vi "Autonomous Independentold.vi"() -> ()   [LabVIEW 2014]
doc: "This VI is called when autonomous begins, and will automatically be terminated when autonomous ends. You can carry out timed or sensor driven robot movement independently without needing to return to the caller."
uses:
  <vilib>/Rock Robotics/WPI/Joystick/WPI_JoystickGetSetRefNum.vi
  <vilib>/Rock Robotics/Network Tables/SD Write Numeric Array.vi
  <vilib>/Rock Robotics/WPI/RobotDrive/WPI_RobotDriveMecanumDrive_Cartesian.vi
  <vilib>/Rock Robotics/Network Tables/SD Write String.vi
panel:
  in  "error in":errorcluster
  out "error out":errorcluster
  in  "error in":errorcluster
  out "error out":errorcluster
  out "error out":errorcluster
  in  "error in":errorcluster
  in  "stop":bool
  out "Current Movement, for debugging":T1 {"Z Joystick Value" scale=-1.0..1.0; "Y Joystick Value" scale=1.0..-1.0; "X Joystick Value" scale=-1.0..1.0}
  in  "Array of robot movements":T2(array[cluster]) {"Z Joystick Value" scale=-1.0..1.0; "Y Joystick Value" scale=1.0..-1.0; "X Joystick Value" scale=-1.0..1.0}
  # "Be sure to right-click and choose Data Operations>>Make Current Value default if you want to save the array values with the VI"
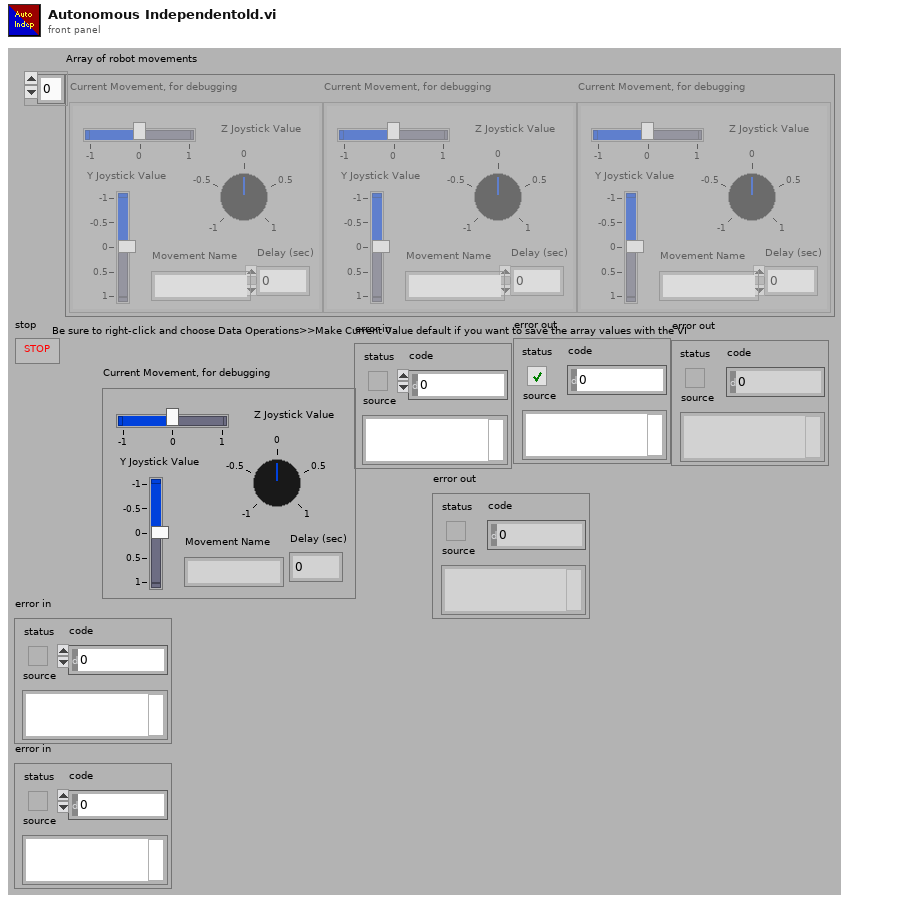
[diagram p1: front panel]
types:
  T1 = cluster{"X Joystick Value":dbl, "Y Joystick Value":dbl, "Z Joystick Value":dbl, "Delay (sec)":dbl, "Movement Name":string}
  T2 = cluster{"X Joystick Value":dbl, "Y Joystick Value":dbl, "Z Joystick Value":dbl, "Delay (sec)":dbl, "Movement Name":string}[]
  T3 = typedef "WPI_JoystickDevRef.ctl" = cluster{"Device":T4}
  T4 = typedef "WPI_JoystickDeviceEnum.ctl" = enum16{"USB 0", "USB 1", "USB 2", "USB 3", "USB 4", "USB 5"}
  T5 = typedef "WPI_RobotDriveDevRef.ctl" = cluster{"DevStatus":errorcluster, "Motors[]":T6[], "Square Inputs":bool, "Max Output":dbl}
  T6 = typedef "WPI_MotorControlDeviceRef.ctl" = cluster{"DeviceStatus":errorcluster, "Type":T7, "PWM":cluster{"Controller":T8, "PWM Channel":T9, "DeadBand":T10}, "CAN":cluster{"Device Number":u8, "Control Mode":T11, "Semaphore":T12, "Max Vout":dbl, "TalonSRX Control Mode":T13}, "Invert":bool, "TransformRef":T14, "InvTransformRef":T14}
  T7 = typedef "WPI_MotorControlType.ctl" = enum16{"PWM", "CAN", "CANTalonSRX"}
  T8 = typedef "FPGA_TypedefDigitalModule.ctl" = enum16{"Controller 1"}
  T9 = typedef "FPGA_DIOPWMChannel.ctl" = enum8{"PWM 0", "PWM 1", "PWM 2", "PWM 3", "PWM 4", "PWM 5", "PWM 6", "PWM 7", "PWM 8", "PWM 9", "PWM MXP 0", "PWM MXP 1", "PWM MXP 2", "PWM MXP 3", "PWM MXP 4", "PWM MXP 5", "PWM MXP 6", "PWM MXP 7", "PWM MXP 8", "PWM MXP 9", "Invalid"}
  T10 = typedef "WPI_PWMDeadband.ctl" = cluster{"Name":string, "maxPositivePwm":i32, "minPositivePwm":i32, "centerPwm":i32, "maxNegativePwm":i32, "minNegativePwm":i32, "angularRange":u16}
  T11 = typedef "WPI_CANJaguar_ControlMode.ctl" = enum8{"Percent VBus", "Current", "Speed", "Position", "Voltage"}
  T12 = typedef "Semaphore RefNum" = refnum<k1>
  T13 = typedef "WPI_CANTalonSRX_APIControlMode.ctl" = enum8{"Percent VBus", "Speed", "Position", "Slave", "Unchanged / Invalid"}
  T14 = typedef "WPI_PWMTransform_ConPane.ctl" = refnum<vi>
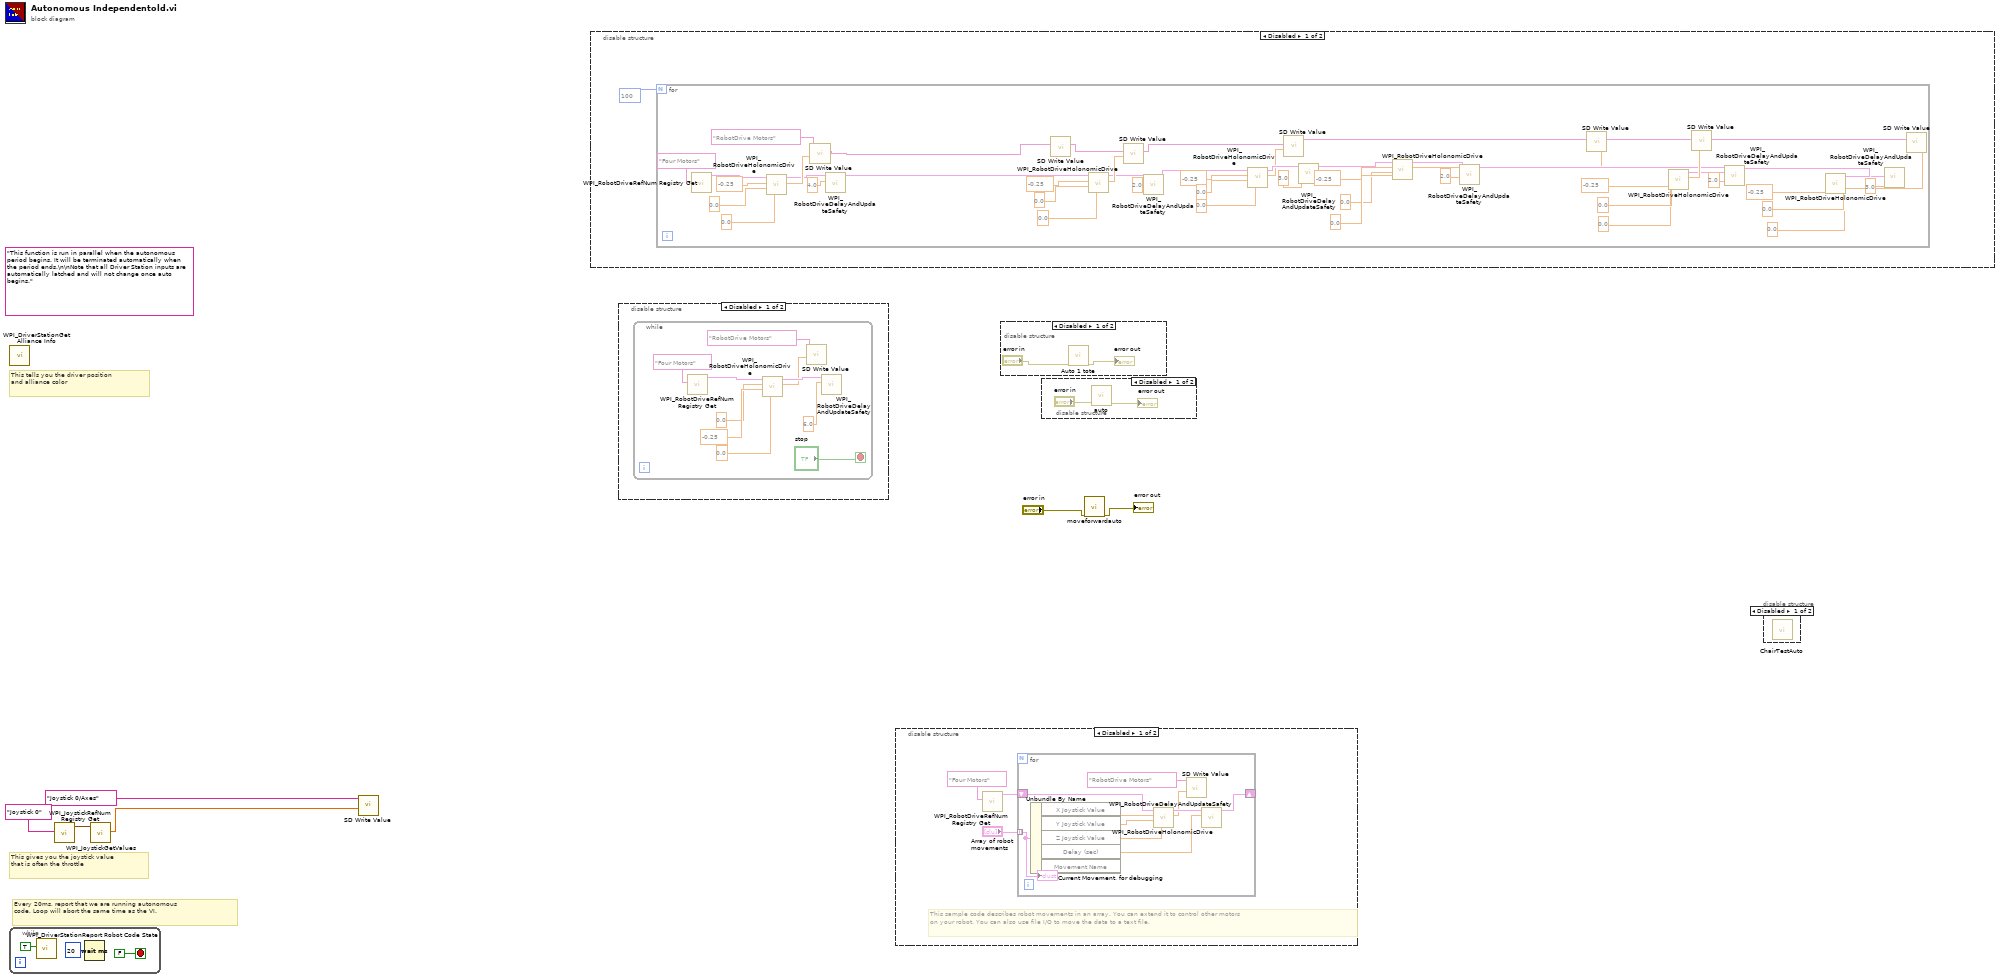
[diagram p0: block diagram]
diagram:
  (unwired) "This function is run in parallel when the autonomous period begins. It will be terminated automatically when the period ends.\n\nNote that all Driver Station inputs are automatically latched and will not change once auto begins."
  # "Every 20ms, report that we are running autonomous\ncode. Loop will abort the same time as the VI."
  # "This gives you the joystick value\nthat is often the throttle"
  # "This tells you the driver position\nand alliance color"
  n1 = while {
    stop <- FALSE stop-if-true
    n2 = call <vilib>:"WPI_DriverStationReport Robot Code State.vi"("Autonomous"=TRUE) -> ()  [unwired: 10 in, 1 out]
    n3 = Wait (ms)(milliseconds to wait=u32 20) -> ()  [unwired: 1 out]
  }
  n4 = call <vilib>:"WPI_DriverStationGet Alliance Info.vi"() -> ()  [unwired: 12 out]
  n5 = call <vilib>:"WPI_JoystickRefNum Registry Get.vi"("refnum name"="Joystick 0") -> ("JoystickDevRef"=w5:T3)  [unwired: 1 in, 9 out]
  n6 = call <vilib>:"WPI_JoystickGetValues.vi"("JoystickDevRef"=w5) -> ("Axes"=w3:dbl[])  [unwired: 6 in, 4 out]
  n7 = call-poly <vilib>:"SD Write Value.vi"("Numeric Array"=w3, "Name"="Joystick 0/Axes") -> ()  [unwired: 8 in, 2 out]
  n8 = disable-structure shown="Disabled" {
    frame Disabled {
      n9 = for {
        N: 100 -> [_]
        n10 = call <vilib>:"WPI_RobotDriveRefNum Registry Get.vi"("refnum name"="Four Motors") -> ("RobotDriveDevRef"=w29:T5)  [unwired: 1 in, 9 out]
        n11 = call-poly <vilib>:"WPI_RobotDriveHolonomicDrive.vi"("Rotation"=0.0, "Y"=0.0 ("X axis value"), "X"=-0.25 ("X axis value"), "RobotDriveDevRef"=w29) -> ("Motor Values"=w33:dbl[], "RobotDriveDevRef"=w23:T5)  [unwired: 5 in, 1 out]
        n12 = call-poly <vilib>:"SD Write Value.vi"("Numeric Array"=w33, "Name"="RobotDrive Motors") -> ("Table Prefix out"=w11:string)  [unwired: 8 in, 1 out]
        n13 = call <vilib>:"WPI_RobotDriveDelayAndUpdateSafety.vi"("Delay (s)"=4.0, "RobotDriveDevRef"=w23) -> ("RobotDriveDevRef 2"=w12:T5)  [unwired: 8 in, 1 out]
        n14 = call-poly <vilib>:"SD Write Value.vi"("Table Prefix"=w11) -> ("Table Prefix out"=w14:string)  [unwired: 9 in, 1 out]
        n15 = call-poly <vilib>:"WPI_RobotDriveHolonomicDrive.vi"("Rotation"=0.0, "Y"=0.0 ("X axis value"), "X"=-0.25 ("X axis value"), "RobotDriveDevRef"=w12) -> ("Motor Values"=w34:dbl[], "RobotDriveDevRef"=w24:T5)  [unwired: 5 in, 1 out]
        n16 = call-poly <vilib>:"SD Write Value.vi"("Numeric Array"=w34, "Table Prefix"=w14) -> ("Table Prefix out"=w13:string)  [unwired: 8 in, 1 out]
        n17 = call <vilib>:"WPI_RobotDriveDelayAndUpdateSafety.vi"("Delay (s)"=2.0, "RobotDriveDevRef"=w24) -> ("RobotDriveDevRef 2"=w25:T5)  [unwired: 8 in, 1 out]
        n18 = call-poly <vilib>:"WPI_RobotDriveHolonomicDrive.vi"("Rotation"=0.0 ("X axis value"), "Y"=0.0 ("X axis value"), "X"=-0.25 ("X axis value"), "RobotDriveDevRef"=w25) -> ("Motor Values"=w35:dbl[], "RobotDriveDevRef"=w37:T5)  [unwired: 5 in, 1 out]
        n19 = call-poly <vilib>:"SD Write Value.vi"("Numeric Array"=w35, "Table Prefix"=w13) -> ("Table Prefix out"=w44:string)  [unwired: 8 in, 1 out]
        n20 = call <vilib>:"WPI_RobotDriveDelayAndUpdateSafety.vi"("Delay (s)"=3.0, "RobotDriveDevRef"=w37) -> ("RobotDriveDevRef 2"=w38:T5)  [unwired: 8 in, 1 out]
        n21 = call-poly <vilib>:"WPI_RobotDriveHolonomicDrive.vi"("Rotation"=0.0, "Y"=0.0, "X"=-0.25, "RobotDriveDevRef"=w38) -> ("Motor Values"=w45:dbl[], "RobotDriveDevRef"=w42:T5)  [unwired: 5 in, 1 out]
        n22 = call <vilib>:"WPI_RobotDriveDelayAndUpdateSafety.vi"("Delay (s)"=2.0, "RobotDriveDevRef"=w42) -> ("RobotDriveDevRef 2"=w46:T5)  [unwired: 8 in, 1 out]
        n23 = call-poly <vilib>:"SD Write Value.vi"("Numeric Array"=w45, "Table Prefix"=w44) -> ("Table Prefix out"=w56:string)  [unwired: 8 in, 1 out]
        n24 = call-poly <vilib>:"WPI_RobotDriveHolonomicDrive.vi"("Rotation"=0.0, "Y"=0.0, "X"=-0.25, "RobotDriveDevRef"=w46) -> ("Motor Values"=w58:dbl[], "RobotDriveDevRef"=w50:T5)  [unwired: 5 in, 1 out]
        n25 = call-poly <vilib>:"SD Write Value.vi"("Numeric Array"=w58, "Table Prefix"=w56) -> ("Table Prefix out"=w60:string)  [unwired: 8 in, 1 out]
        n26 = call <vilib>:"WPI_RobotDriveDelayAndUpdateSafety.vi"("Delay (s)"=2.0, "RobotDriveDevRef"=w50) -> ("RobotDriveDevRef 2"=w57:T5)  [unwired: 8 in, 1 out]
        n27 = call-poly <vilib>:"WPI_RobotDriveHolonomicDrive.vi"("Rotation"=0.0, "Y"=0.0, "X"=-0.25, "RobotDriveDevRef"=w57) -> ("Motor Values"=w59:dbl[], "RobotDriveDevRef"=w54:T5)  [unwired: 5 in, 1 out]
        n28 = call <vilib>:"WPI_RobotDriveDelayAndUpdateSafety.vi"("Delay (s)"=3.0, "RobotDriveDevRef"=w54) -> ()  [unwired: 8 in, 2 out]
        n29 = call-poly <vilib>:"SD Write Value.vi"("Numeric Array"=w59, "Table Prefix"=w60) -> ()  [unwired: 8 in, 2 out]
      }
    }
    frame Enabled {
    }
  }
  n30 = disable-structure shown="Disabled" {
    frame Disabled {
      n31 = while {
        stop <- "stop" stop-if-true
        n32 = call <vilib>:"WPI_RobotDriveRefNum Registry Get.vi"("refnum name"="Four Motors") -> ("RobotDriveDevRef"=w64:T5)  [unwired: 1 in, 9 out]
        n33 = call-poly <vilib>:"WPI_RobotDriveHolonomicDrive.vi"("Rotation"=0.0, "Y"=-0.25 ("X axis value"), "X"=0.0 ("X axis value"), "RobotDriveDevRef"=w64) -> ("Motor Values"=w62:dbl[], "RobotDriveDevRef"=w67:T5)  [unwired: 5 in, 1 out]
        n34 = call-poly <vilib>:"SD Write Value.vi"("Numeric Array"=w62, "Name"="RobotDrive Motors") -> ()  [unwired: 8 in, 2 out]
        n35 = call <vilib>:"WPI_RobotDriveDelayAndUpdateSafety.vi"("Delay (s)"=6.0, "RobotDriveDevRef"=w67) -> ()  [unwired: 8 in, 2 out]
      }
    }
    frame Enabled {
    }
  }
  n36 = disable-structure shown="Disabled" {
    frame Disabled {
      # "This sample code describes robot movements in an array. You can extend it to control other motors\non your robot. You can also use file I/O to move the data to a text file."
      n37 = call <vilib>:"WPI_RobotDriveRefNum Registry Get.vi"("refnum name"="Four Motors") -> ("RobotDriveDevRef"=w72:T5)  [unwired: 1 in, 9 out]
      n38 = for {
        shift-right: [w80] -> _
        shift-left: w72 -> [w81]
        tunnel: "Array of robot movements" -> [w76] mode=indexing
        n39 = Unbundle By Name(w76) -> ("X Joystick Value"=w79:dbl, "Y Joystick Value"=w78:dbl, "Z Joystick Value"=w75:dbl, "Delay (sec)"=w77:dbl)  [unwired: 1 out]
        n40 = call-poly <vilib>:"WPI_RobotDriveHolonomicDrive.vi"("Rotation"=w75, "Y"=w78, "X"=w79, "RobotDriveDevRef"=w81) -> ("Motor Values"=w74:dbl[], "RobotDriveDevRef"=w82:T5)  [unwired: 5 in, 1 out]
        n41 = call-poly <vilib>:"SD Write Value.vi"("Numeric Array"=w74, "Name"="RobotDrive Motors") -> ()  [unwired: 8 in, 2 out]
        n42 = call <vilib>:"WPI_RobotDriveDelayAndUpdateSafety.vi"("Delay (s)"=w77, "RobotDriveDevRef"=w82) -> ("RobotDriveDevRef 2"=w80:T5)  [unwired: 8 in, 1 out]
        "Current Movement, for debugging" <- w76
      }
    }
    frame Enabled {
    }
  }
  n43 = disable-structure shown="Disabled" {
    frame Disabled {
      n44 = call "Auto 1 tote.vi"("error in (no error)"="error in") -> ("error out"=→"error out":errorcluster)  [unwired: 10 in]
    }
    frame Enabled {
    }
  }
  n45 = disable-structure shown="Disabled" {
    frame Disabled {
      n46 = call "auto.vi"("error in (no error)"="error in") -> ("error out"=→"error out":errorcluster)  [unwired: 10 in]
    }
    frame Enabled {
    }
  }
  n47 = call "moveforwardauto.vi"("error in (no error)"="error in") -> ("error out"=→"error out":errorcluster)  [unwired: 10 in]
  n48 = disable-structure shown="Disabled" {
    frame Disabled {
      n49 = call "ChairTestAuto.vi"() -> ()  [unwired: 12 in]
    }
    frame Enabled {
    }
  }
